vi "niRFUtil RFHS Util Library Info.vi"(11 "error in (no error)":errorcluster) -> (4 "info":string, 6 "version":string, 8 "version":u32 format="%08x", 10 "path":path, 14 "AVX support":bool, 15 "error out":errorcluster)   [LabVIEW 2015, in "niRFUtil.lvlib"]
uses:
  niRFUtil.lvlib
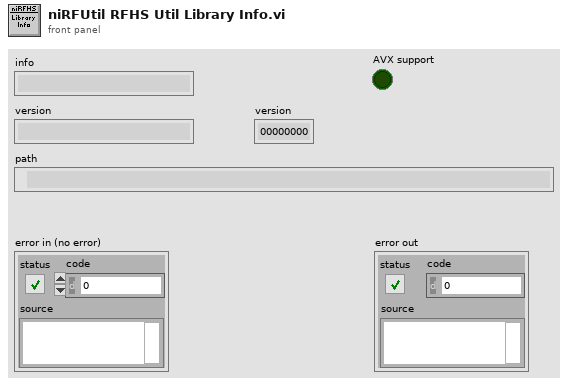
[diagram p1: front panel]
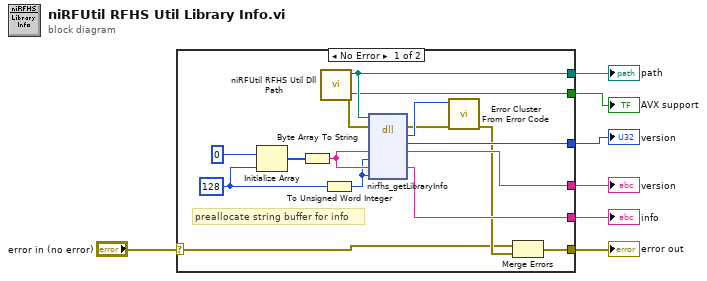
[diagram p0: block diagram]
diagram:
  n1 = case shown="No Error" "error in (no error)" {
    selector: "error in (no error)" -> [w10 w24]
    tunnel: [w12 w24] -> w6
    tunnel: [w19 _] -> w5
    tunnel: [w18 _] -> w4
    tunnel: [w14 _] -> w3
    tunnel: [w9 _] -> w2
    tunnel: [w8 _] -> w1
    frame No Error {
      w16 = 128 ("dimension size")
      # "preallocate string buffer for info"
      n2 = Initialize Array(u8 0 ("element"), w16) -> (w20:u8[])
      n3 = Byte Array To String(unsigned byte array=w20) -> (string=w17:string)
      n4 = call "niRFUtil RFHS Util Dll Path.vi"() -> ("error out"=w13:errorcluster, "Path"=w9:path, "AVX support"=w8:bool)  [unwired: 7 in, 2 out]
      n5 = To Unsigned Word Integer(number=w16) -> (unsigned 16bit integer=w15:u16)
      n6 = dll-call lib="M:/RfProtocols/RFmx/DLLs/niRFHS/trunk/2.0/dist/win32U/niRFHS_generic.*" fn="nirfhs_getLibraryInfo"(path in=w9, error in=w13, "versionString"=w17, "versionStringBufSize"=w15, "info"=w17, "infoBufSize"=w15) -> (error out=w22:errorcluster, "return type"=w23:i32, "version"=w19:u32, "versionString"=w14:string, "info"=w18:string)  [unwired: 4 in, 1 out]
      n7 = call <vilib>:"Error Cluster From Error Code.vi"("error in (no error)"=w22, "error code (0)"=w23) -> ("error out"=w11:errorcluster)  [unwired: 7 in]
      n8 = Merge Errors(w10, w11) -> (w12:errorcluster)
    }
    frame Error {
    }
  }
  "error out" <- w6
  "info" <- w4
  "version" <- w5
  "version" <- w3
  "path" <- w2
  "AVX support" <- w1
